vi "SetpointsToTCP.vi"(10 "remote port or service name":u16=10001, 11 "address":string="192.168.1.11") -> (0 "error out":errorcluster, 3 "TCP Connected?":bool)   [LabVIEW 2011]
uses:
  2-RIO/2 Typedefs/setpoints to boat.ctl
  2-RIO/2 Typedefs/sail setpt.ctl
  2-RIO/2 Typedefs/rudder angle.ctl
  2-RIO/2 Typedefs/generalized actuator status.ctl
  2-RIO/2 Typedefs/indicator LED.ctl
  2-RIO/2 Globals/2 Global.vi
panel:
  out "Output Array":u8[](array[numeric])
  out "Setpoints to boat out":T1
  in  "VI Stop":bool
  # "This is the Set-Points to TCP writer.\n\nThis vi reads the global variable setpoints and passes them through to the TCP connection.\n\nTODO: make it actually work. Connection to the global variable seems a bit glitchy, as does the TCP connection."
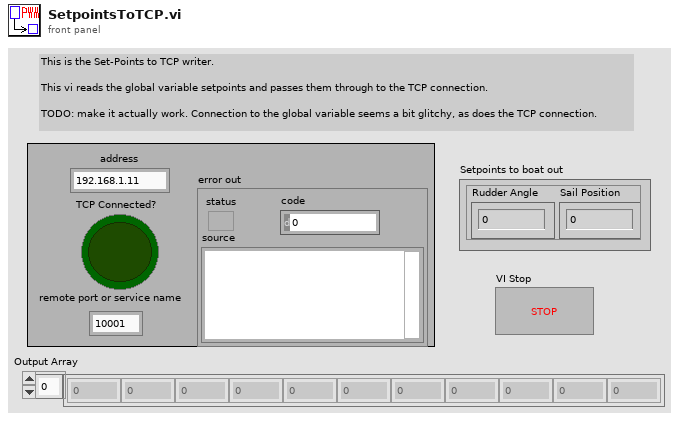
[diagram p1: front panel]
types:
  T1 = typedef "setpoints to boat.ctl" = cluster{"Sail Position":T2, "Rudder Angle":T3}
  T2 = typedef "sail setpt.ctl" = dbl
  T3 = typedef "rudder angle.ctl" = dbl
  T4 = typedef "generalized actuator status.ctl" = cluster{"Actuator Connected":T5}
  T5 = typedef "indicator LED.ctl" = bool
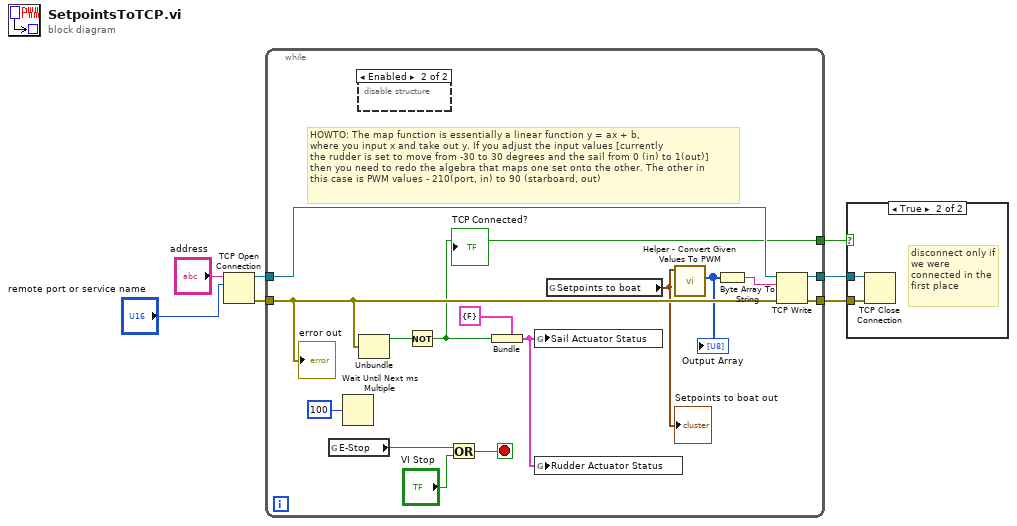
[diagram p0: block diagram]
diagram:
  n1 = TCP Open Connection(address="address", remote port or service name="remote port or service name") -> (connection ID=w3:refnum<k5>, error out=w5:errorcluster)  [unwired: 3 in]
  n2 = while {
    tunnel: w5 -> [w19]
    tunnel: [w22] -> w4
    tunnel: w3 -> [w21]
    tunnel: [w20] -> w2
    tunnel: [w8] -> w1
    stop <- w15 stop-if-true
    # "HOWTO: The map function is essentially a linear function y = ax + b,\nwhere you input x and take out y. If you adjust the input values [currently\nthe rudder is set to move from -30 to 30 degrees and the sail from 0 (in) to 1(out)]\nthen you need to redo the algebra that maps one set onto the other. The other in\nthis case is PWM values - 210(port, in) to 90 (starboard, out)"
    n3 = global read "2 Global.vi" "E-Stop"() -> (w13:bool)
    n4 = Wait Until Next ms Multiple(millisecond multiple=u32 100) -> ()  [unwired: 1 out]
    n5 = disable-structure shown="Enabled" {
      frame Disabled {
      }
      frame Enabled {
      }
    }
    n6 = Unbundle(w19) -> ("status"=w18:bool)  [unwired: 2 out]
    n7 = Not(x=w18) -> (.not. x?=w8:bool)
    "TCP Connected?" <- w8
    n8 = Or(x=w13, y="VI Stop") -> (x .or. y?=w15:bool)
    n9 = Bundle(cluster=T4 {"Actuator Connected"=FALSE} ("Sail Actuator Status"), "Actuator Connected"=w8) -> (w11:T4)
    n10 = global write "2 Global.vi" "Sail Actuator Status"(w11) -> ()
    n11 = global write "2 Global.vi" "Rudder Actuator Status"(w11) -> ()
    n12 = global read "2 Global.vi" "Setpoints to boat"() -> (w9:T1)
    "Setpoints to boat out" <- w9
    n13 = call "Helper - Convert Given Values To PWM.vi"("Setpoints to boat"=w9) -> ("Output Array, integers"=w10:u8[])  [unwired: 9 in, 1 out]
    "Output Array" <- w10
    n14 = Byte Array To String(unsigned byte array=w10) -> (string=w17:string)
    n15 = TCP Write(connection ID=w21, data in=w17, error in (no error)=w19) -> (connection ID out=w20:refnum<k5>, error out=w22:errorcluster)  [unwired: 1 in, 1 out]
    "error out" <- w19
  }
  n16 = case shown="True" w1 {
    tunnel: w4 -> [_ w24]
    tunnel: w2 -> [_ w23]
    frame False {
    }
    frame True {
      # "disconnect only if we were connected in the first place"
      n17 = TCP Close Connection(connection ID=w23, error in (no error)=w24) -> ()  [unwired: 1 in, 2 out]
    }
  }
